vi "IRD_M_E.vi"() -> ()   [LabVIEW 2017]
panel:
  out "Counter Value":T1(graph)
  in  "Stop VI":bool
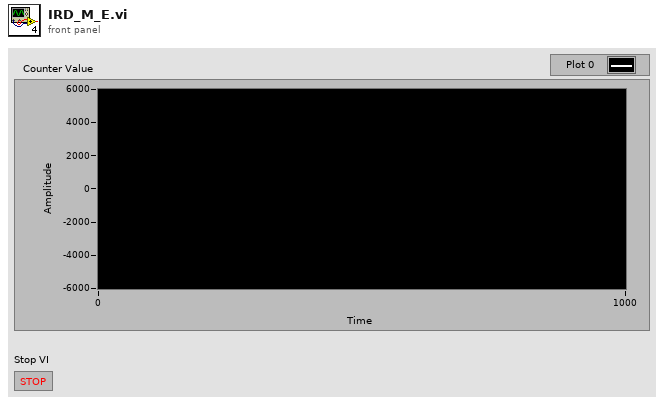
[diagram p1: front panel]
types:
  T1 = cluster{"Counter Value":dbl, "Counter Value":dbl}
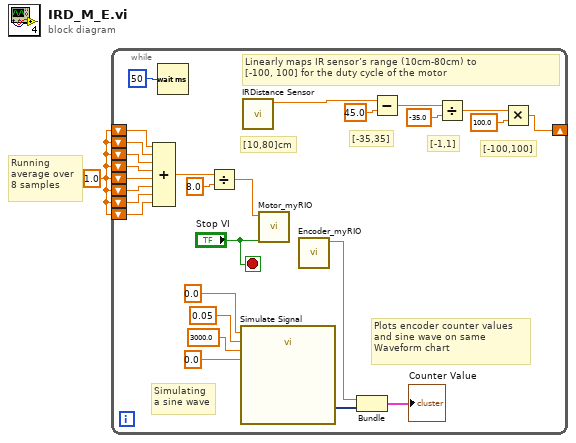
[diagram p0: block diagram]
diagram:
  w1 = 1.0
  # "Running\naverage over \n8 samples"
  n1 = while {
    shift-right: [w5] -> _
    shift-left: w1 -> [w28]
    shift-left: w1 -> [w27]
    shift-left: w1 -> [w26]
    shift-left: w1 -> [w25]
    shift-left: w1 -> [w24]
    shift-left: w1 -> [w23]
    shift-left: w1 -> [w20]
    shift-left: w1 -> [w19]
    stop <- "Stop VI" stop-if-true
    # "[10,80]cm"
    # "[-100,100]"
    # "[-1,1]"
    # "[-35,35]"
    # "Linearly maps IR sensor’s range (10cm-80cm) to \n[-100, 100] for the duty cycle of the motor"
    # "Plots encoder counter values \nand sine wave on same \nWaveform chart"
    # "Simulating\na sine wave"
    n2 = Compound Arithmetic op=ADD(w19, w20, w28, w27, w26, w25, w24, w23) -> (w22:dbl)
    n3 = Wait (ms)(milliseconds to wait=u32 50) -> ()  [unwired: 1 out]
    n4 = Divide(x=w22, y=8.0) -> (x/y=w3:dbl)
    n5 = call "Simulate Signal"("Offset"=0.0, "Frequency"=0.05, "Amplitude"=3000.0, "Phase"=0.0) -> ("Sine"=w17:dynamicdata)  [unwired: 10 in, 1 out]
    n6 = call "IRDistance Sensor.vi"() -> ("interpolation value"=w11:dbl)  [unwired: 11 in]
    n7 = call "Motor_myRIO.vi"("Stop VI"="Stop VI", "Duty Cycle (-100 to +100)"=w3) -> ()  [unwired: 10 in]
    n8 = call "Encoder_myRIO.vi"() -> ("Counter Value"=w2:dbl)  [unwired: 10 in, 1 out]
    n9 = Bundle("Counter Value"=w2, "Sine"=w17) -> (→"Counter Value":cluster{"Counter Value":dbl, "Sine":dynamicdata})  [unwired: 1 in]
    n10 = Subtract(x=w11, y=45.0) -> (x-y=w9:dbl)
    n11 = Divide(x=w9, y=-35.0) -> (x/y=w7:dbl)
    n12 = Multiply(x=w7, y=100.0) -> (x*y=w5:dbl)
  }
